vi "libssh2_session_banner_set.vi"(8 "error in (no error)":errorcluster, 10 "banner":string, 11 "session":T1) -> (0 "error out":errorcluster)   [LabVIEW 2013, in "libssh2.lvlib"]
doc: "Set the banner that will be sent to the server when a session is established."
uses:
  libssh2.lvlib
  Session Refnum.ctl
  Not A Session.vi
  <vilib>/Utility/error.llb/Error Cluster From Error Code.vi
  Global Settings.vi
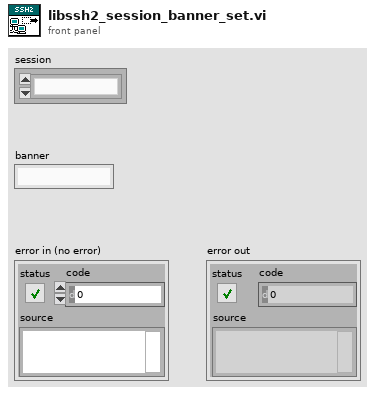
[diagram p1: front panel]
types:
  T1 = typedef "libssh2.lvlib/Session Refnum.ctl" = refnum<k1>
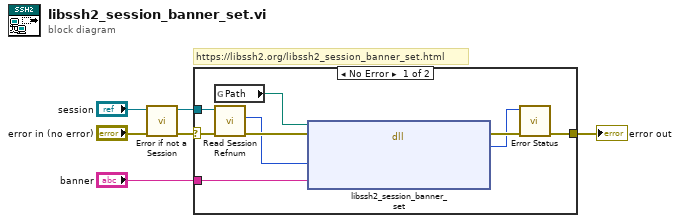
[diagram p0: block diagram]
diagram:
  # "https://libssh2.org/libssh2_session_banner_set.html"
  n1 = call "Error if not a Session.vi"("error in (no error)"="error in (no error)", "session"="session") -> ("error out"=w4:errorcluster, "session out"=w2:T1)  [unwired: 8 in]
  n2 = case shown="No Error" w4 {
    selector: w4 -> [w14 w16]
    tunnel: [w8 w16] -> w6
    tunnel: w2 -> [w13 _]
    tunnel: "banner" -> [w9 _]
    frame No Error {
      n3 = global read "Global Settings.vi" "Path"() -> (w10:path)
      n4 = call "Read Session Refnum.vi"("error in (no error)"=w14, "session"=w13) -> ("error out"=w12:errorcluster, "LIBSSH2_SESSION*"=w11:u64)  [unwired: 5 in, 3 out]
      n5 = dll-call lib="?" fn="libssh2_session_banner_set"(path in=w10, error in=w12, "session"=w11, "banner"=w9) -> (error out=w15:errorcluster, "return value"=w7:i32)  [unwired: 3 in, 1 out]
      n6 = call "Error Status.vi"("error in (no error)"=w15, "return value"=w7) -> ("error out"=w8:errorcluster)  [unwired: 8 in, 1 out]
    }
    frame Error {
    }
  }
  "error out" <- w6
